vi "Return_Data.vi"(8 "error in (no error)":errorcluster caption="entrée d'erreur (pas d'erreur)", 11 "Class Instrument Patterm_Matching en entrée":refnum<class "Class Instrument Patterm_Matching.lvclass">) -> (0 "error out":errorcluster caption="sortie d'erreur", 2 "Data_Json":string, 3 "Class Instrument Patterm_Matching en sortie":refnum<class "Class Instrument Patterm_Matching.lvclass">)   [LabVIEW 2020, in "Library Instrument & Equipement.lvlib" / "Library Instruments.lvlib" / "Class Instrument Patterm_Matching.lvclass"]
uses:
  Class Instrument Patterm_Matching.lvclass
  Class Instrument Patterm_Matching.lvclass/Class Instrument Patterm_Matching.ctl
  JSON API/Variant JSON/Variant to JSON.vi
  JSON API/JSON Value/Get Item by name array.vi
  JSON API/JSON Value/JSON Value.lvclass
  JSON API/Get Polymorphic/JSON GetSet.lvlib
  JSON API/Variant JSON/Variant JSON.lvlib
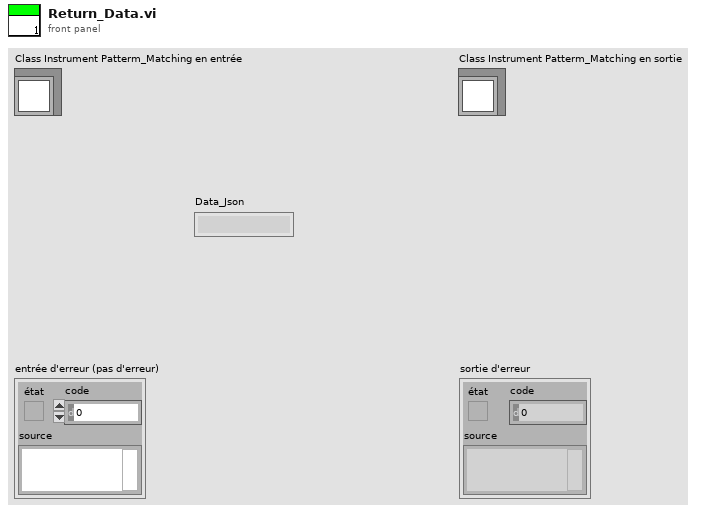
[diagram p1: front panel]
types:
  T1 = cluster{"Result Test":bool, "Result Value":string}
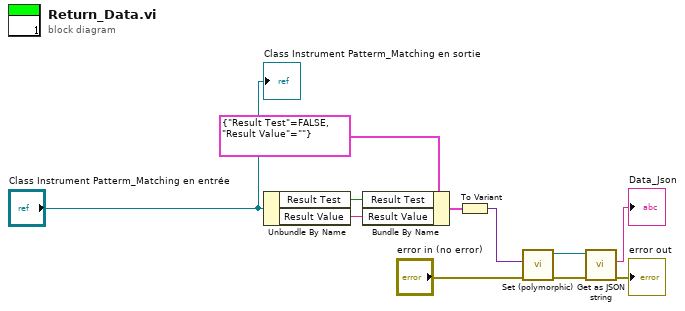
[diagram p0: block diagram]
diagram:
  n1 = Unbundle By Name("Class Instrument Patterm_Matching en entrée") -> ("Result Test"=w3:bool, "Result Value"=w2:string)
  n2 = Bundle By Name(cluster=T1 {"Result Test"=FALSE, "Result Value"=""}, "Result Test"=w3, "Result Value"=w2) -> (w1:T1)
  n3 = To Variant(anything=w1) -> (Variant=w9:variant)
  n4 = call-poly "Set (polymorphic).vi"("error in (no error)"="error in (no error)", "Variant"=w9) -> ("error out"=w10:errorcluster, "JSON Value out"=w11:refnum<class "JSON Value.lvclass">)  [unwired: 8 in]
  n5 = call "Get as JSON string.vi"("error in (no error)"=w10, "JSON Value in"=w11) -> ("error out"=→"error out":errorcluster, "<JSON>"=→"Data_Json":string)  [unwired: 8 in]
  "Class Instrument Patterm_Matching en sortie" <- "Class Instrument Patterm_Matching en entrée"
